vi "OnDataChange.vi"(0 "Device in":refnum<class "Device.lvclass">, 1 "DataExchange":T1, 3 "error in (no error)":errorcluster) -> (7 "Device out":refnum<class "Device.lvclass">, 10 "error out":errorcluster)   [LabVIEW 2020, in "Device.lvlib" / "Device.lvclass"]
uses:
  Device.lvclass
  DataExchange.ctl
  Interface/DataListener/DataListener.lvclass
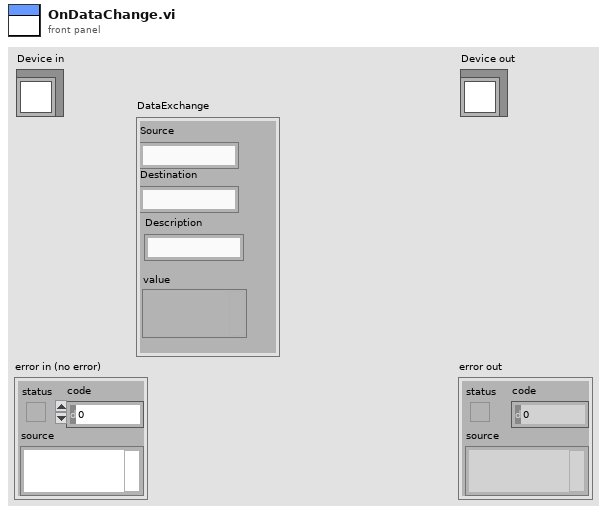
[diagram p1: front panel]
types:
  T1 = typedef "DataListener.lvclass/DataExchange.ctl" = cluster{"Source":string, "Destination":string, "Description":string, "value":variant}
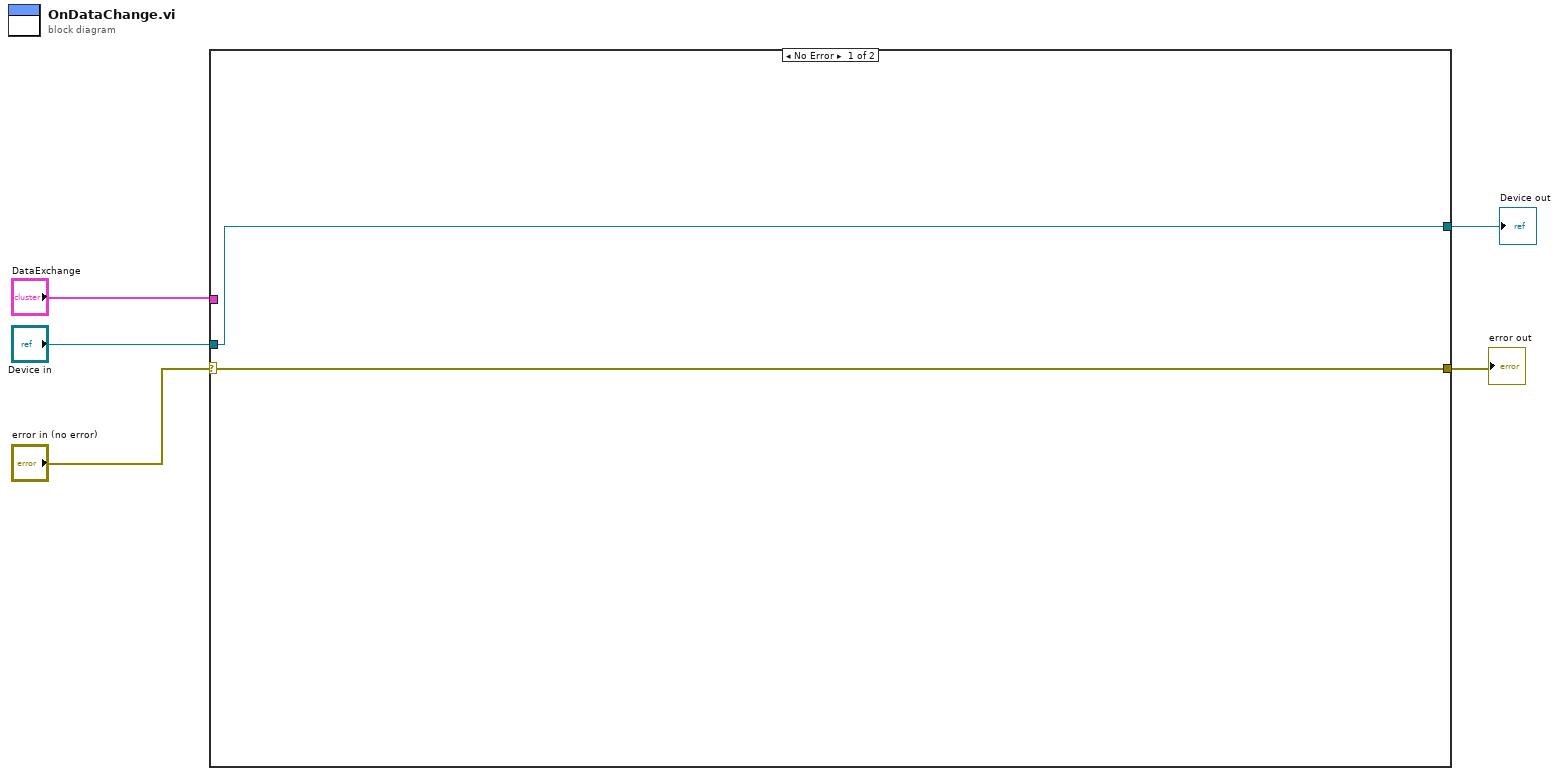
[diagram p0: block diagram]
diagram:
  n1 = case shown="No Error" "error in (no error)" {
    selector: "error in (no error)" -> [w6 w9]
    tunnel: [w6 w9] -> w4
    tunnel: "Device in" -> [w7 w8]
    tunnel: [w7 w8] -> w5
    tunnel: "DataExchange" -> [_ _]
    frame No Error {
    }
    frame Error {
    }
  }
  "error out" <- w4
  "Device out" <- w5
